vi "TCPFrameProcess.vi"() -> ()   [LabVIEW 2021]
panel:
  in  "input arrray":u8[](array[numeric])
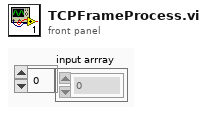
[diagram p1: front panel]
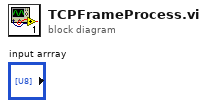
[diagram p0: block diagram]
diagram:
